vi "signal sampling digital.vi"() -> ()   [LabVIEW 2018]
uses:
  <vilib>/Waveform/DWDTOps.llb/DWDT Analog to Digital.vi
panel:
  in  "stop":bool
  out "Waveform Graph":waveform(dbl)(graph)
  out "Digital Waveform Graph":digitalwaveform(graph)
  out "digital waveform":digitalwaveform(waveform)={"t0"=timestamp(0 s since 1904-01-01), "dt"=0.0, "Y"={"transitions"=[], "data"=[]}, "error"={"status"=FALSE, "code"=37421928, "source"=""}}
  in  "amplitude":dbl=1.0 format="%0.2p"
  in  "frequency":dbl=10.0 format="%0.2p"
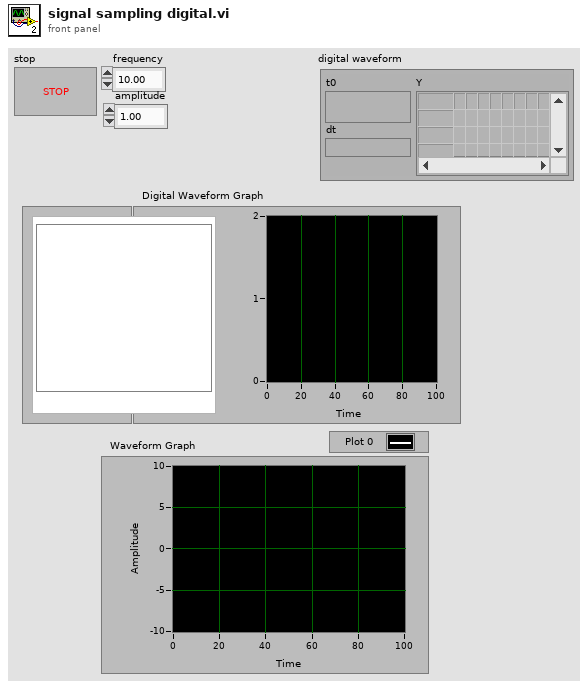
[diagram p1: front panel]
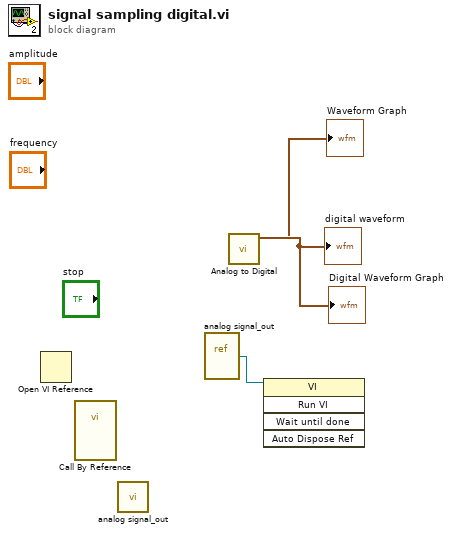
[diagram p0: block diagram]
diagram:
  n1 = Open VI Reference() -> ()  [unwired: 6 in, 2 out]
  n2 = call-by-ref "?"() -> ()  [unwired: 12 in, 3 out]
  n3 = call "analog signal_out.vi"() -> ()  [unwired: 10 in, 1 out]
  n4 = vi-ref "analog signal_out.vi"() -> (w1:refnum<vi>)
  n5 = call-poly <vilib>:"Analog to Digital.vi"("analog waveform"="Waveform Graph") -> ("digital waveform"=→"digital waveform" →"Digital Waveform Graph":digitalwaveform)  [unwired: 7 in, 3 out]
  n6 = invoke class="VI" method="Run VI"(reference=w1) -> ()  [unwired: 4 in, 5 out]
